vi "Read CPU Done.vi"(8 "error in (no error)":errorcluster, 11 "Simple UI in":refnum<class "Simple UI.lvclass">) -> (0 "error out":errorcluster, 2 "CPU Done":refnum<user-event>, 3 "Simple UI out":refnum<class "Simple UI.lvclass">)   [LabVIEW 2020, in "Simple UI.lvlib" / "Simple UI.lvclass"]
uses:
  Simple UI.lvclass
  Simple UI.lvclass/Simple UI.ctl
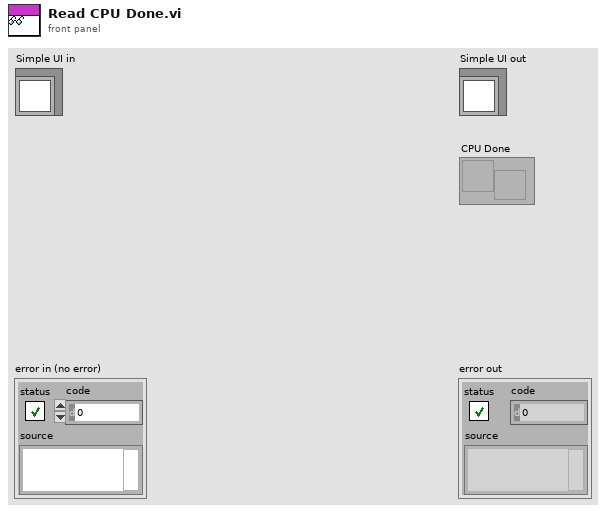
[diagram p1: front panel]
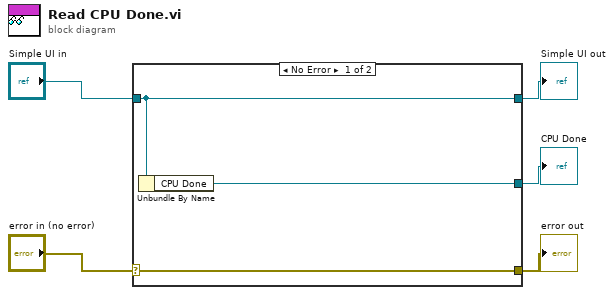
[diagram p0: block diagram]
diagram:
  n1 = case shown="No Error" "error in (no error)" {
    selector: "error in (no error)" -> [w8 w9]
    tunnel: [w8 w9] -> w4
    tunnel: [w7 w10] -> w2
    tunnel: "Simple UI in" -> [w7 w10]
    tunnel: [w6 _] -> w1
    frame No Error {
      n2 = Unbundle By Name(w7) -> ("CPU Done"=w6:refnum<user-event>)
    }
    frame Error {
    }
  }
  "error out" <- w4
  "Simple UI out" <- w2
  "CPU Done" <- w1
